vi "GeoData.vi"() -> ()   [LabVIEW 2017] (continued)
H1\n66625\t20177\tTopeka\tKS\tShawnee County\tH1\n66409\t20177\tBerryton\tKS\tShawnee County\tH1\n66536\t20177\tSaint marys\tKS\tShawnee County\tH1\n66524\t20177\tOverbrook\tKS\tShawnee County\tH1\n66614\t20177\tTopeka\tKS\tShawnee County\tH1\n66636\t20177\tTopeka\tKS\tShawnee County\tH1\n66667\t20177\tTopeka\tKS\tShawnee County\tH1\n66624\t20177\tTopeka\tKS\tShawnee County\tH1\n66420\t20177\tDover\tKS\tShawnee County\tH1\n66609\t20177\tTopeka\tKS\tShawnee County\tH1\n66615\t20177\tTopeka\tKS\tShawnee County\tH1\n66603\t20177\tTopeka\tKS\tShawnee County\tH1\n66546\t20177\tWakarusa\tKS\tShawnee County\tH1\n66647\t20177\tTopeka\tKS\tShawnee County\tH1\n66542\t20177\tTecumseh\tKS\tShawnee County\tH1\n66608\t20177\tTopeka\tKS\tShawnee County\tH1\n66612\t20177\tTopeka\tKS\tShawnee County\tH1\n66621\t20177\tTopeka\tKS\tShawnee County\tH1\n66620\t20177\tTopeka\tKS\tShawnee County\tH1\n66626\t20177\tTopeka\tKS\tShawnee County\tH1\n66533\t20177\tRossville\tKS\tShawnee County\tH1\n66604\t20177\tTopeka\tKS\tShawnee County\tH1\n66606\t20177\tTopeka\tKS\tShawnee County\tH1\n66675\t20177\tTopeka\tKS\tShawnee County\tH1\n66699\t20177\tTopeka\tKS\tShawnee County\tH1\n66402\t20177\tAuburn\tKS\tShawnee County\tH1\n66618\t20177\tTopeka\tKS\tShawnee County\tH1\n66607\t20177\tTopeka\tKS\tShawnee County\tH1\n66616\t20177\tTopeka\tKS\tShawnee County\tH1\n66683\t20177\tTopeka\tKS\tShawnee County\tH1\n66629\t20177\tTopeka\tKS\tShawnee County\tH1\n66622\t20177\tTopeka\tKS\tShawnee County\tH1\n67757\t20179\tSelden\tKS\tSheridan County\tH1\n67738\t20179\tGrinnell\tKS\tSheridan County\tH1\n67740\t20179\tHoxie\tKS\tSheridan County\tH1\n67753\t20179\tRexford\tKS\tSheridan County\tH1\n67732\t20181\tBrewster\tKS\tSherman County\tH1\n67741\t20181\tKanorado\tKS\tSherman County\tH1\n67735\t20181\tGoodland\tKS\tSherman County\tH1\n67733\t20181\tEdson\tKS\tSherman County\tH1\n67762\t20181\tWeskan\tKS\tSherman County\tH1\n66967\t20183\tSmith center\tKS\tSmith County\tH1\n67474\t20183\tPortis\tKS\tSmith County\tH1\n66941\t20183\tEsbon\tKS\tSmith County\tH1\n66952\t20183\tLebanon\tKS\tSmith County\tH1\n66951\t20183\tKensington\tKS\tSmith County\tH1\n66932\t20183\tAthol\tKS\tSmith County\tH1\n67628\t20183\tCedar\tKS\tSmith County\tH1\n67437\t20183\tDowns\tKS\tSmith County\tH1\n67638\t20183\tGaylord\tKS\tSmith County\tH1\n67526\t20185\tEllinwood\tKS\tStafford County\tH1\n67578\t20185\tStafford\tKS\tStafford County\tH1\n67545\t20185\tHudson\tKS\tStafford County\tH1\n67576\t20185\tSt john\tKS\tStafford County\tH1\n67530\t20185\tGreat bend\tKS\tStafford County\tH1\n67557\t20185\tMacksville\tKS\tStafford County\tH1\n67583\t20185\tTuron\tKS\tStafford County\tH1\n67855\t20187\tJohnson\tKS\tStanton County\tH1\n67862\t20187\tManter\tKS\tStanton County\tH1\n67880\t20187\tUlysses\tKS\tStanton County\tH1\n67878\t20187\tSyracuse\tKS\tStanton County\tH1\n67951\t20189\tHugoton\tKS\tStevens County\tH1\n67954\t20189\tRolla\tKS\tStevens County\tH1\n67953\t20189\tRichfield\tKS\tStevens County\tH1\n67952\t20189\tMoscow\tKS\tStevens County\tH1\n67026\t20191\tClearwater\tKS\tSumner County\tH1\n67022\t20191\tCaldwell\tKS\tSumner County\tH1\n67119\t20191\tOxford\tKS\tSumner County\tH1\n67110\t20191\tMulvane\tKS\tSumner County\tH1\n67049\t20191\tFreeport\tKS\tSumner County\tH1\n67152\t20191\tWellington\tKS\tSumner County\tH1\n67051\t20191\tGeuda springs\tKS\tSumner County\tH1\n67013\t20191\tBelle plaine\tKS\tSumner County\tH1\n67031\t20191\tConway springs\tKS\tSumner County\tH1\n67004\t20191\tArgonia\tKS\tSumner County\tH1\n67140\t20191\tSouth haven\tKS\tSumner County\tH1\n67120\t20191\tPeck\tKS\tSumner County\tH1\n67105\t20191\tMilan\tKS\tSumner County\tH1\n67146\t20191\tUdall\tKS\tSumner County\tH1\n67018\t20191\tBluff city\tKS\tSumner County\tH1\n67106\t20191\tMilton\tKS\tSumner County\tH1\n67103\t20191\tMayfield\tKS\tSumner County\tH1\n67118\t20191\tNorwich\tKS\tSumner County\tH1\n67748\t20193\tOakley\tKS\tThomas County\tH1\n67757\t20193\tSelden\tKS\tThomas County\tH1\n67732\t20193\tBrewster\tKS\tThomas County\tH1\n67764\t20193\tWinona\tKS\tThomas County\tH1\n67743\t20193\tLevant\tKS\tThomas County\tH1\n67747\t20193\tMonument\tKS\tThomas County\tH1\n67701\t20193\tColby\tKS\tThomas County\tH1\n67734\t20193\tGem\tKS\tThomas County\tH1\n67753\t20193\tRexford\tKS\tThomas County\tH1\n67656\t20195\tOgallah\tKS\tTrego County\tH1\n67752\t20195\tQuinter\tKS\tTrego County\tH1\n67584\t20195\tUtica\tKS\tTrego County\tH1\n67572\t20195\tRansom\tKS\tTrego County\tH1\n67672\t20195\tWakeeney\tKS\tTrego County\tH1\n67521\t20195\tBrownell\tKS\tTrego County\tH1\n67637\t20195\tEllis\tKS\tTrego County\tH1\n67631\t20195\tCollyer\tKS\tTrego County\tH1\n66431\t20197\tHarveyville\tKS\tWabaunsee County\tH1\n66610\t20197\tTopeka\tKS\tWabaunsee County\tH1\n66401\t20197\tAlma\tKS\tWabaunsee County\tH1\n66547\t20197\tWamego\tKS\tWabaunsee County\tH1\n66834\t20197\tAlta vista\tKS\tWabaunsee County\tH1\n66501\t20197\tMc farland\tKS\tWabaunsee County\tH1\n66502\t20197\tManhattan\tKS\tWabaunsee County\tH1\n66413\t20197\tBurlingame\tKS\tWabaunsee County\tH1\n66536\t20197\tSaint marys\tKS\tWabaunsee County\tH1\n66614\t20197\tTopeka\tKS\tWabaunsee County\tH1\n66407\t20197\tBelvue\tKS\tWabaunsee County\tH1\n66846\t20197\tCouncil grove\tKS\tWabaunsee County\tH1\n66615\t20197\tTopeka\tKS\tWabaunsee County\tH1\n66526\t20197\tPaxico\tKS\tWabaunsee County\tH1\n66423\t20197\tEskridge\tKS\tWabaunsee County\tH1\n66507\t20197\tMaple hill\tKS\tWabaunsee County\tH1\n67861\t20199\tLeoti\tKS\tWallace County\tH1\n67758\t20199\tSharon springs\tKS\tWallace County\tH1\n67761\t20199\tWallace\tKS\tWallace County\tH1\n67762\t20199\tWeskan\tKS\tWallace County\tH1\n66943\t20201\tGreenleaf\tKS\tWashington County\tH1\n66953\t20201\tLinn\tKS\tWashington County\tH1\n66933\t20201\tBarnes\tKS\tWashington County\tH1\n66946\t20201\tHollenberg\tKS\tWashington County\tH1\n66548\t20201\tWaterville\tKS\tWashington County\tH1\n66955\t20201\tMahaska\tKS\tWashington County\tH1\n66960\t20201\tNarka\tKS\tWashington County\tH1\n66945\t20201\tHanover\tKS\tWashington County\tH1\n66937\t20201\tClifton\tKS\tWashington County\tH1\n66412\t20201\tBremen\tKS\tWashington County\tH1\n66968\t20201\tWashington\tKS\tWashington County\tH1\n66958\t20201\tMorrowville\tKS\tWashington County\tH1\n66962\t20201\tPalmer\tKS\tWashington County\tH1\n66938\t20201\tClyde\tKS\tWashington County\tH1\n66944\t20201\tHaddam\tKS\tWashington County\tH1\n67861\t20203\tLeoti\tKS\tWichita County\tH1\n67863\t20203\tMarienthal\tKS\tWichita County\tH1\n66736\t20205\tFredonia\tKS\tWilson County\tH1\n66776\t20205\tThayer\tKS\tWilson County\tH1\n66757\t20205\tNeodesha\tKS\tWilson County\tH1\n66714\t20205\tBenedict\tKS\tWilson County\tH1\n66717\t20205\tBuffalo\tKS\tWilson County\tH1\n67047\t20205\tFall river\tKS\tWilson County\tH1\n66710\t20205\tAltoona\tKS\tWilson County\tH1\n66777\t20205\tToronto\tKS\tWilson County\tH1\n67335\t20205\tCherryvale\tKS\tWilson County\tH1\n66720\t20205\tChanute\tKS\tWilson County\tH1\n66749\t20207\tIola\tKS\tWoodson County\tH1\n66870\t20207\tVirgil\tKS\tWoodson County\tH1\n66783\t20207\tYates center\tKS\tWoodson County\tH1\n66736\t20207\tFredonia\tKS\tWoodson County\tH1\n66761\t20207\tPiqua\tKS\tWoodson County\tH1\n66748\t20207\tHumboldt\tKS\tWoodson County\tH1\n66852\t20207\tGridley\tKS\tWoodson County\tH1\n66758\t20207\tNeosho falls\tKS\tWoodson County\tH1\n66717\t20207\tBuffalo\tKS\tWoodson County\tH1\n66777\t20207\tToronto\tKS\tWoodson County\tH1\n66115\t20209\tKansas city\tKS\tWyandotte County\tH6\n66104\t20209\tKansas city\tKS\tWyandotte County\tH6\n66103\t20209\tKansas city\tKS\tWyandotte County\tH6\n66117\t20209\tKansas city\tKS\tWyandotte County\tH6\n66106\t20209\tKansas city\tKS\tWyandotte County\tH6\n66216\t20209\tShawnee\tKS\tWyandotte County\tH6\n66119\t20209\tKansas city\tKS\tWyandotte County\tH6\n66217\t20209\tShawnee\tKS\tWyandotte County\tH6\n66102\t20209\tKansas city\tKS\tWyandotte County\tH6\n66048\t20209\tLeavenworth\tKS\tWyandotte County\tH6\n66007\t20209\tBasehor\tKS\tWyandotte County\tH6\n66118\t20209\tKansas city\tKS\tWyandotte County\tH6\n66112\t20209\tKansas city\tKS\tWyandotte County\tH6\n66160\t20209\tKansas city\tKS\tWyandotte County\tH6\n66012\t20209\tBonner springs\tKS\tWyandotte County\tH6\n66109\t20209\tKansas city\tKS\tWyandotte County\tH6\n66111\t20209\tKansas city\tKS\tWyandotte County\tH6\n66101\t20209\tKansas city\tKS\tWyandotte County\tH6\n66105\t20209\tKansas city\tKS\tWyandotte County\tH6\n42129\t21001\tEdmonton\tKY\tAdair County\tH1\n42642\t21001\tRussell springs\tKY\tAdair County\tH1\n42728\t21001\tColumbia\tKY\tAdair County\tH1\n42715\t21001\tBreeding\tKY\tAdair County\tH1\n42741\t21001\tGlens fork\tKY\tAdair County\tH1\n42539\t21001\tLiberty\tKY\tAdair County\tH1\n42743\t21001\tGreensburg\tKY\tAdair County\tH1\n42742\t21001\tGradyville\tKY\tAdair County\tH1\n42733\t21001\tElk horn\tKY\tAdair County\tH1\n42718\t21001\tCampbellsville\tKY\tAdair County\tH1\n42753\t21001\tKnifley\tKY\tAdair County\tH1\n42528\t21001\tDunnville\tKY\tAdair County\tH1\n42720\t21001\tCane valley\tKY\tAdair County\tH1\n42133\t21003\tFountain run\tKY\tAllen County\tH1\n42134\t21003\tFranklin\tKY\tAllen County\tH1\n42122\t21003\tAlvaton\tKY\tAllen County\tH1\n42164\t21003\tScottsville\tKY\tAllen County\tH1\n42153\t21003\tHolland\tKY\tAllen County\tH1\n42120\t21003\tAdolphus\tKY\tAllen County\tH1\n40046\t21005\tMount eden\tKY\tAnderson County\tH1\n40012\t21005\tChaplin\tKY\tAnderson County\tH1\n40078\t21005\tWillisburg\tKY\tAnderson County\tH1\n40601\t21005\tFrankfort\tKY\tAnderson County\tH1\n40342\t21005\tLawrenceburg\tKY\tAnderson County\tH1\n40076\t21005\tWaddy\tKY\tAnderson County\tH1\n40372\t21005\tSalvisa\tKY\tAnderson County\tH1\n42024\t21007\tBarlow\tKY\tBallard County\tH1\n42053\t21007\tKevil\tKY\tBallard County\tH1\n42087\t21007\tWickliffe\tKY\tBallard County\tH1\n42022\t21007\tBandana\tKY\tBallard County\tH1\n42056\t21007\tLa center\tKY\tBallard County\tH1\n42060\t21007\tLovelaceville\tKY\tBallard County\tH1\n42133\t21009\tFountain run\tKY\tBarren County\tH1\n42131\t21009\tEtoile\tKY\tBarren County\tH1\n42171\t21009\tSmiths grove\tKY\tBarren County\tH1\n42166\t21009\tSummer shade\tKY\tBarren County\tH1\n42749\t21009\tHorse cave\tKY\tBarren County\tH1\n42152\t21009\tHiseville\tKY\tBarren County\tH1\n42123\t21009\tAustin\tKY\tBarren County\tH1\n42130\t21009\tEighty eight\tKY\tBarren County\tH1\n42127\t21009\tCave city\tKY\tBarren County\tH1\n42157\t21009\tMount hermon\tKY\tBarren County\tH1\n42154\t21009\tKnob lick\tKY\tBarren County\tH1\n42141\t21009\tGlasgow\tKY\tBarren County\tH1\n42156\t21009\tLucas\tKY\tBarren County\tH1\n42160\t21009\tPark city\tKY\tBarren County\tH1\n42746\t21009\tHardyville\tKY\tBarren County\tH1\n40358\t21011\tOlympia\tKY\tBath County\tH1\n40311\t21011\tCarlisle\tKY\tBath County\tH1\n40353\t21011\tMount sterling\tKY\tBath County\tH1\n40346\t21011\tMeans\tKY\tBath County\tH1\n40334\t21011\tHope\tKY\tBath County\tH1\n40351\t21011\tMorehead\tKY\tBath County\tH1\n41041\t21011\tFlemingsburg\tKY\tBath County\tH1\n40371\t21011\tSalt lick\tKY\tBath County\tH1\n40360\t21011\tOwingsville\tKY\tBath County\tH1\n40374\t21011\tSharpsburg\tKY\tBath County\tH1\n40322\t21011\tFrenchburg\tKY\tBath County\tH1\n40958\t21013\tKettle island\tKY\tBell County\tH1\n40930\t21013\tDewitt\tKY\tBell County\tH1\n40977\t21013\tPineville\tKY\tBell County\tH1\n40955\t21013\tIngram\tKY\tBell County\tH1\n40845\t21013\tHulen\tKY\tBell County\tH1\n40856\t21013\tMiracle\tKY\tBell County\tH1\n40939\t21013\tFourmile\tKY\tBell County\tH1\n40988\t21013\tStoney fork\tKY\tBell County\tH1\n40813\t21013\tCalvin\tKY\tBell County\tH1\n40902\t21013\tArjay\tKY\tBell County\tH1\n40965\t21013\tMiddlesboro\tKY\tBell County\tH1\n40913\t21013\tBeverly\tKY\tBell County\tH1\n40940\t21013\tFrakes\tKY\tBell County\tH1\n41048\t21015\tHebron\tKY\tBoone County\tH1\n45275\t21015\tCincinnati\tKY\tBoone County\tH1\n41025\t21015\tErlanger\tKY\tBoone County\tH1\n41091\t21015\tUnion\tKY\tBoone County\tH1\n41092\t21015\tVerona\tKY\tBoone County\tH1\n41005\t21015\tBurlington\tKY\tBoone County\tH1\n41018\t21015\tErlanger\tKY\tBoone County\tH1\n41030\t21015\tCrittenden\tKY\tBoone County\tH1\n41042\t21015\tFlorence\tKY\tBoone County\tH1\n41094\t21015\tWalton\tKY\tBoone County\tH1\n41080\t21015\tPetersburg\tKY\tBoone County\tH1\n41051\t21015\tIndependence\tKY\tBoone County\tH1\n41022\t21015\tFlorence\tKY\tBoone County\tH1\n40311\t21017\tCarlisle\tKY\tBourbon County\tH1\n41031\t21017\tCynthiana\tKY\tBourbon County\tH1\n40353\t21017\tMount sterling\tKY\tBourbon County\tH1\n40357\t21017\tNorth middletown\tKY\tBourbon County\tH1\n40324\t21017\tGeorgetown\tKY\tBourbon County\tH1\n40511\t21017\tLexington\tKY\tBourbon County\tH1\n40361\t21017\tParis\tKY\tBourbon County\tH1\n40516\t21017\tLexington\tKY\tBourbon County\tH1\n40348\t21017\tMillersburg\tKY\tBourbon County\tH1\n40374\t21017\tSharpsburg\tKY\tBourbon County\tH1\n41102\t21019\tAshland\tKY\tBoyd County\tH1\n41132\t21019\tDenton\tKY\tBoyd County\tH1\n41101\t21019\tAshland\tKY\tBoyd County\tH1\n41168\t21019\tRush\tKY\tBoyd County\tH1\n41129\t21019\tCatlettsburg\tKY\tBoyd County\tH1\n41230\t21019\tLouisa\tKY\tBoyd County\tH1\n41105\t21019\tAshland\tKY\tBoyd County\tH1\n40468\t21021\tPerryville\tKY\tBoyle County\tH1\n40464\t21021\tParksville\tKY\tBoyle County\tH1\n40440\t21021\tJunction city\tKY\tBoyle County\tH1\n40422\t21021\tDanville\tKY\tBoyle County\tH1\n40452\t21021\tMitchellsburg\tKY\tBoyle County\tH1\n40330\t21021\tHarrodsburg\tKY\tBoyle County\tH1\n40328\t21021\tGravel switch\tKY\tBoyle County\tH1\n41043\t21023\tFoster\tKY\tBracken County\tH1\n41044\t21023\tGermantown\tKY\tBracken County\tH1\n41002\t21023\tAugusta\tKY\tBracken County\tH1\n41034\t21023\tDover\tKY\tBracken County\tH1\n41004\t21023\tBrooksville\tKY\tBracken County\tH1\n41064\t21023\tMount olivet\tKY\tBracken County\tH1\n41040\t21023\tFalmouth\tKY\tBracken County\tH1\n41061\t21023\tMilford\tKY\tBracken County\tH1\n41339\t21025\tJackson\tKY\tBreathitt County\tH1\n41721\t21025\tBuckhorn\tKY\tBreathitt County\tH1\n41390\t21025\tWhick\tKY\tBreathitt County\tH1\n41745\t21025\tGays creek\tKY\tBreathitt County\tH1\n41311\t21025\tBeattyville\tKY\tBreathitt County\tH1\n41317\t21025\tClayhole\tKY\tBreathitt County\tH1\n41314\t21025\tBooneville\tKY\tBreathitt County\tH1\n41385\t21025\tVancleve\tKY\tBreathitt County\tH1\n41366\t21025\tRousseau\tKY\tBreathitt County\tH1\n41727\t21025\tChavies\tKY\tBreathitt County\tH1\n41301\t21025\tCampton\tKY\tBreathitt County\tH1\n41364\t21025\tRicetown\tKY\tBreathitt County\tH1\n41310\t21025\tBays\tKY\tBreathitt County\tH1\n41348\t21025\tLost creek\tKY\tBreathitt County\tH1\n40146\t21027\tIrvington\tKY\tBreckinridge County\tH1\n40161\t21027\tRhodelia\tKY\tBreckinridge County\tH1\n40157\t21027\tPayneville\tKY\tBreckinridge County\tH1\n42712\t21027\tBig clifty\tKY\tBreckinridge County\tH1\n40140\t21027\tGarfield\tKY\tBreckinridge County\tH1\n40170\t21027\tStephensport\tKY\tBreckinridge County\tH1\n40153\t21027\tMc quady\tKY\tBreckinridge County\tH1\n40111\t21027\tCloverport\tKY\tBreckinridge County\tH1\n40152\t21027\tMc daniels\tKY\tBreckinridge County\tH1\n40144\t21027\tHarned\tKY\tBreckinridge County\tH1\n42343\t21027\tFordsville\tKY\tBreckinridge County\tH1\n40175\t21027\tVine grove\tKY\tBreckinridge County\tH1\n42754\t21027\tLeitchfield\tKY\tBreckinridge County\tH1\n40171\t21027\tUnion star\tKY\tBreckinridge County\tH1\n40142\t21027\tGuston\tKY\tBreckinridge County\tH1\n40145\t21027\tHudson\tKY\tBreckinridge County\tH1\n40176\t21027\tWebster\tKY\tBreckinridge County\tH1\n40119\t21027\tFalls of rough\tKY\tBreckinridge County\tH1\n40115\t21027\tCuster\tKY\tBreckinridge County\tH1\n40143\t21027\tHardinsburg\tKY\tBreckinridge County\tH1\n40178\t21027\tWestview\tKY\tBreckinridge County\tH1\n40229\t21029\tLouisville\tKY\tBullitt County\tH1\n40207\t21029\tLouisville\tKY\tBullitt County\tH1\n40272\t21029\tLouisville\tKY\tBullitt County\tH1\n40166\t21029\tShepherdsville\tKY\tBullitt County\tH1\n40150\t21029\tLebanon junction\tKY\tBullitt County\tH1\n40177\t21029\tWest point\tKY\tBullitt County\tH1\n40110\t21029\tClermont\tKY\tBullitt County\tH1\n40047\t21029\tMount washington\tKY\tBullitt County\tH1\n40129\t21029\tHillview\tKY\tBullitt County\tH1\n40071\t21029\tTaylorsville\tKY\tBullitt County\tH1\n40165\t21029\tShepherdsville\tKY\tBullitt County\tH1\n40013\t21029\tCoxs creek\tKY\tBullitt County\tH1\n40109\t21029\tBrooks\tKY\tBullitt County\tH1\n40299\t21029\tLouisville\tKY\tBullitt County\tH1\n42101\t21031\tBowling green\tKY\tButler County\tH1\n42339\t21031\tDunmor\tKY\tButler County\tH1\n42288\t21031\tWoodbury\tKY\tButler County\tH1\n42721\t21031\tCaneyville\tKY\tButler County\tH1\n42219\t21031\tDunbar\tKY\tButler County\tH1\n42276\t21031\tRussellville\tKY\tButler County\tH1\n42256\t21031\tLewisburg\tKY\tButler County\tH1\n42333\t21031\tCromwell\tKY\tButler County\tH1\n42273\t21031\tRochester\tKY\tButler County\tH1\n42252\t21031\tJetson\tKY\tButler County\tH1\n42275\t21031\tRoundhill\tKY\tButler County\tH1\n42320\t21031\tBeaver dam\tKY\tButler County\tH1\n42201\t21031\tAberdeen\tKY\tButler County\tH1\n42261\t21031\tMorgantown\tKY\tButler County\tH1\n42211\t21033\tCadiz\tKY\tCaldwell County\tH1\n42411\t21033\tFredonia\tKY\tCaldwell County\tH1\n42445\t21033\tPrinceton\tKY\tCaldwell County\tH1\n42064\t21033\tMarion\tKY\tCaldwell County\tH1\n42408\t21033\tDawson springs\tKY\tCaldwell County\tH1\n42048\t21035\tHardin\tKY\tCalloway County\tH1\n42020\t21035\tAlmo\tKY\tCalloway County\tH1\n42054\t21035\tKirksey\tKY\tCalloway County\tH1\n42025\t21035\tBenton\tKY\tCalloway County\tH1\n42049\t21035\tHazel\tKY\tCalloway County\tH1\n42076\t21035\tNew concord\tKY\tCalloway County\tH1\n42071\t21035\tMurray\tKY\tCalloway County\tH1\n42040\t21035\tFarmington\tKY\tCalloway County\tH1\n42066\t21035\tMayfield\tKY\tCalloway County\tH1\n42036\t21035\tDexter\tKY\tCalloway County\tH1\n41074\t21037\tDayton\tKY\tCampbell County\tH1\n41071\t21037\tNewport\tKY\tCampbell County\tH1\n41076\t21037\tNewport\tKY\tCampbell County\tH1\n41001\t21037\tAlexandria\tKY\tCampbell County\tH1\n41059\t21037\tMelbourne\tKY\tCampbell County\tH1\n41075\t21037\tFort thomas\tKY\tCampbell County\tH1\n41007\t21037\tCalifornia\tKY\tCampbell County\tH1\n41085\t21037\tSilver grove\tKY\tCampbell County\tH1\n41072\t21037\tNewport\tKY\tCampbell County\tH1\n41099\t21037\tNewport\tKY\tCampbell County\tH1\n41006\t21037\tButler\tKY\tCampbell County\tH1\n41073\t21037\tBellevue\tKY\tCampbell County\tH1\n42039\t21039\tFancy farm\tKY\tCarlisle County\tH1\n42035\t21039\tCunningham\tKY\tCarlisle County\tH1\n42023\t21039\tBardwell\tKY\tCarlisle County\tH1\n42021\t21039\tArlington\tKY\tCarlisle County\tH1\n42069\t21039\tMelber\tKY\tCarlisle County\tH1\n40075\t21041\tTurners station\tKY\tCarroll County\tH1\n41045\t21041\tGhent\tKY\tCarroll County\tH1\n40006\t21041\tBedford\tKY\tCarroll County\tH1\n41098\t21041\tWorthville\tKY\tCarroll County\tH1\n41083\t21041\tSanders\tKY\tCarroll County\tH1\n41008\t21041\tCarrollton\tKY\tCarroll County\tH1\n40045\t21041\tMilton\tKY\tCarroll County\tH1\n40011\t21041\tCampbellsburg\tKY\tCarroll County\tH1\n41121\t21043\tArgillite\tKY\tCarter County\tH1\n41132\t21043\tDenton\tKY\tCarter County\tH1\n41143\t21043\tGrayson\tKY\tCarter County\tH1\n41171\t21043\tSandy hook\tKY\tCarter County\tH1\n40351\t21043\tMorehead\tKY\tCarter County\tH1\n41180\t21043\tWebbville\tKY\tCarter County\tH1\n41173\t21043\tSoldier\tKY\tCarter County\tH1\n41144\t21043\tGreenup\tKY\tCarter County\tH1\n41179\t21043\tVanceburg\tKY\tCarter County\tH1\n41168\t21043\tRush\tKY\tCarter County\tH1\n41141\t21043\tGarrison\tKY\tCarter County\tH1\n41142\t21043\tGrahn\tKY\tCarter County\tH1\n41164\t21043\tOlive hill\tKY\tCarter County\tH1\n41230\t21043\tLouisa\tKY\tCarter County\tH1\n41146\t21043\tHitchins\tKY\tCarter County\tH1\n40437\t21045\tHustonville\tKY\tCasey County\tH1\n40442\t21045\tKings mountain\tKY\tCasey County\tH1\n40009\t21045\tBradfordsville\tKY\tCasey County\tH1\n40484\t21045\tStanford\tKY\tCasey County\tH1\n40489\t21045\tWaynesburg\tKY\tCasey County\tH1\n42642\t21045\tRussell springs\tKY\tCasey County\tH1\n42541\t21045\tMiddleburg\tKY\tCasey County\tH1\n42728\t21045\tColumbia\tKY\tCasey County\tH1\n40464\t21045\tParksville\tKY\tCasey County\tH1\n42539\t21045\tLiberty\tKY\tCasey County\tH1\n42565\t21045\tWindsor\tKY\tCasey County\tH1\n42544\t21045\tNancy\tKY\tCasey County\tH1\n42566\t21045\tYosemite\tKY\tCasey County\tH1\n42733\t21045\tElk horn\tKY\tCasey County\tH1\n42553\t21045\tScience hill\tKY\tCasey County\tH1\n42516\t21045\tBethelridge\tKY\tCasey County\tH1\n40328\t21045\tGravel switch\tKY\tCasey County\tH1\n42528\t21045\tDunnville\tKY\tCasey County\tH1\n42215\t21047\tCerulean\tKY\tChristian County\tH1\n42266\t21047\tPembroke\tKY\tChristian County\tH1\n42236\t21047\tHerndon\tKY\tChristian County\tH1\n42232\t21047\tGracey\tKY\tChristian County\tH1\n42262\t21047\tOak grove\tKY\tChristian County\tH1\n42408\t21047\tDawson springs\tKY\tChristian County\tH1\n42254\t21047\tLa fayette\tKY\tChristian County\tH1\n42220\t21047\tElkton\tKY\tChristian County\tH1\n42217\t21047\tCrofton\tKY\tChristian County\tH1\n42453\t21047\tSaint charles\tKY\tChristian County\tH1\n42240\t21047\tHopkinsville\tKY\tChristian County\tH1\n42442\t21047\tNortonville\tKY\tChristian County\tH1\n42241\t21047\tHopkinsville\tKY\tChristian County\tH1\n42286\t21047\tTrenton\tKY\tChristian County\tH1\n42464\t21047\tWhite plains\tKY\tChristian County\tH1\n40353\t21049\tMount sterling\tKY\tClark County\tH1\n40509\t21049\tLexington\tKY\tClark County\tH1\n40312\t21049\tClay city\tKY\tClark County\tH1\n40391\t21049\tWinchester\tKY\tClark County\tH1\n40392\t21049\tWinchester\tKY\tClark County\tH1\n40515\t21049\tLexington\tKY\tClark County\tH1\n40914\t21051\tBig creek\tKY\tClay County\tH1\n40932\t21051\tFall rock\tKY\tClay County\tH1\n40951\t21051\tHima\tKY\tClay County\tH1\n40402\t21051\tAnnville\tKY\tClay County\tH1\n40906\t21051\tBarbourville\tKY\tClay County\tH1\n40972\t21051\tOneida\tKY\tClay County\tH1\n40941\t21051\tGarrard\tKY\tClay County\tH1\n40744\t21051\tLondon\tKY\tClay County\tH1\n40486\t21051\tTyner\tKY\tClay County\tH1\n40741\t21051\tLondon\tKY\tClay County\tH1\n40962\t21051\tManchester\tKY\tClay County\tH1\n40913\t21051\tBeverly\tKY\tClay County\tH1\n40944\t21051\tGoose rock\tKY\tClay County\tH1\n40831\t21051\tHarlan\tKY\tClay County\tH1\n40983\t21051\tSextons creek\tKY\tClay County\tH1\n42602\t21053\tAlbany\tKY\tClinton County\tH1\n42603\t21053\tAlpha\tKY\tClinton County\tH1\n42633\t21053\tMonticello\tKY\tClinton County\tH1\n42717\t21053\tBurkesville\tKY\tClinton County\tH1\n42038\t21055\tEddyville\tKY\tCrittenden County\tH1\n42459\t21055\tSturgis\tKY\tCrittenden County\tH1\n42411\t21055\tFredonia\tKY\tCrittenden County\tH1\n42078\t21055\tSalem\tKY\tCrittenden County\tH1\n42450\t21055\tProvidence\tKY\tCrittenden County\tH1\n42064\t21055\tMarion\tKY\tCrittenden County\tH1\n42037\t21055\tDycusburg\tKY\tCrittenden County\tH1\n42055\t21055\tKuttawa\tKY\tCrittenden County\tH1\n42033\t21055\tCrayne\tKY\tCrittenden County\tH1\n42129\t21057\tEdmonton\tKY\tCumberland County\tH1\n42715\t21057\tBreeding\tKY\tCumberland County\tH1\n42602\t21057\tAlbany\tKY\tCumberland County\tH1\n42759\t21057\tMarrowbone\tKY\tCumberland County\tH1\n42717\t21057\tBurkesville\tKY\tCumberland County\tH1\n42167\t21057\tTompkinsville\tKY\tCumberland County\tH1\n42348\t21059\tHawesville\tKY\tDaviess County\tH1\n42420\t21059\tHenderson\tKY\tDaviess County\tH1\n42302\t21059\tOwensboro\tKY\tDaviess County\tH1\n42327\t21059\tCalhoun\tKY\tDaviess County\tH1\n42301\t21059\tOwensboro\tKY\tDaviess County\tH1\n42351\t21059\tLewisport\tKY\tDaviess County\tH1\n42303\t21059\tOwensboro\tKY\tDaviess County\tH1\n42366\t21059\tPhilpot\tKY\tDaviess County\tH1\n42378\t21059\tWhitesville\tKY\tDaviess County\tH1\n42356\t21059\tMaple mount\tKY\tDaviess County\tH1\n42355\t21059\tMaceo\tKY\tDaviess County\tH1\n42304\t21059\tOwensboro\tKY\tDaviess County\tH1\n42376\t21059\tUtica\tKY\tDaviess County\tH1\n42101\t21061\tBowling green\tKY\tEdmonson County\tH1\n42171\t21061\tSmiths grove\tKY\tEdmonson County\tH1\n42210\t21061\tBrownsville\tKY\tEdmonson County\tH1\n42259\t21061\tMammoth cave\tKY\tEdmonson County\tH1\n42729\t21061\tCub run\tKY\tEdmonson County\tH1\n42721\t21061\tCaneyville\tKY\tEdmonson County\tH1\n42207\t21061\tBee spring\tKY\tEdmonson County\tH1\n42754\t21061\tLeitchfield\tKY\tEdmonson County\tH1\n42275\t21061\tRoundhill\tKY\tEdmonson County\tH1\n42285\t21061\tSweeden\tKY\tEdmonson County\tH1\n42163\t21061\tRocky hill\tKY\tEdmonson County\tH1\n42160\t21061\tPark city\tKY\tEdmonson County\tH1\n41171\t21063\tSandy hook\tKY\tElliott County\tH1\n41149\t21063\tIsonville\tKY\tElliott County\tH1\n40351\t21063\tMorehead\tKY\tElliott County\tH1\n41180\t21063\tWebbville\tKY\tElliott County\tH1\n41472\t21063\tWest liberty\tKY\tElliott County\tH1\n41164\t21063\tOlive hill\tKY\tElliott County\tH1\n40312\t21065\tClay city\tKY\tEstill County\tH1\n40380\t21065\tStanton\tKY\tEstill County\tH1\n40336\t21065\tIrvine\tKY\tEstill County\tH1\n40385\t21065\tWaco\tKY\tEstill County\tH1\n40472\t21065\tRavenna\tKY\tEstill County\tH1\n40503\t21067\tLexington\tKY\tFayette County\tH6\n40575\t21067\tLexington\tKY\tFayette County\tH6\n40512\t21067\tLexington\tKY\tFayette County\tH6\n40578\t21067\tLexington\tKY\tFayette County\tH6\n40509\t21067\tLexington\tKY\tFayette County\tH6\n40324\t21067\tGeorgetown\tKY\tFayette County\tH6\n40544\t21067\tLexington\tKY\tFayette County\tH6\n40536\t21067\tLexington\tKY\tFayette County\tH6\n40577\t21067\tLexington\tKY\tFayette County\tH6\n40580\t21067\tLexington\tKY\tFayette County\tH6\n40391\t21067\tWinchester\tKY\tFayette County\tH6\n40513\t21067\tLexington\tKY\tFayette County\tH6\n40533\t21067\tLexington\tKY\tFayette County\tH6\n40555\t21067\tLexington\tKY\tFayette County\tH6\n40591\t21067\tLexington\tKY\tFayette County\tH6\n40583\t21067\tLexington\tKY\tFayette County\tH6\n40576\t21067\tLexington\tKY\tFayette County\tH6\n40504\t21067\tLexington\tKY\tFayette County\tH6\n40511\t21067\tLexington\tKY\tFayette County\tH6\n40574\t21067\tLexington\tKY\tFayette County\tH6\n40582\t21067\tLexington\tKY\tFayette County\tH6\n40502\t21067\tLexington\tKY\tFayette County\tH6\n40361\t21067\tParis\tKY\tFayette County\tH6\n40517\t21067\tLexington\tKY\tFayette County\tH6\n40515\t21067\tLexington\tKY\tFayette County\tH6\n40516\t21067\tLexington\tKY\tFayette County\tH6\n40514\t21067\tLexington\tKY\tFayette County\tH6\n40588\t21067\tLexington\tKY\tFayette County\tH6\n40505\t21067\tLexington\tKY\tFayette County\tH6\n40356\t21067\tNicholasville\tKY\tFayette County\tH6\n40510\t21067\tLexington\tKY\tFayette County\tH6\n40524\t21067\tLexington\tKY\tFayette County\tH6\n40522\t21067\tLexington\tKY\tFayette County\tH6\n40506\t21067\tLexington\tKY\tFayette County\tH6\n40581\t21067\tLexington\tKY\tFayette County\tH6\n40508\t21067\tLexington\tKY\tFayette County\tH6\n40507\t21067\tLexington\tKY\tFayette County\tH6\n40523\t21067\tLexington\tKY\tFayette County\tH6\n40579\t21067\tLexington\tKY\tFayette County\tH6\n40526\t21067\tLexington\tKY\tFayette County\tH6\n41056\t21069\tMaysville\tKY\tFleming County\tH1\n41093\t21069\tWallingford\tKY\tFleming County\tH1\n41049\t21069\tHillsboro\tKY\tFleming County\tH1\n41081\t21069\tPlummers landing\tKY\tFleming County\tH1\n40351\t21069\tMorehead\tKY\tFleming County\tH1\n41055\t21069\tMayslick\tKY\tFleming County\tH1\n41039\t21069\tEwing\tKY\tFleming County\tH1\n41041\t21069\tFlemingsburg\tKY\tFleming County\tH1\n41037\t21069\tElizaville\tKY\tFleming County\tH1\n41642\t21071\tIvel\tKY\tFloyd County\tH1\n41612\t21071\tBypro\tKY\tFloyd County\tH1\n41651\t21071\tMinnie\tKY\tFloyd County\tH1\n41621\t21071\tDwale\tKY\tFloyd County\tH1\n41631\t21071\tGrethel\tKY\tFloyd County\tH1\n41606\t21071\tBevinsville\tKY\tFloyd County\tH1\n41647\t21071\tMc dowell\tKY\tFloyd County\tH1\n41650\t21071\tMelvin\tKY\tFloyd County\tH1\n41616\t21071\tDavid\tKY\tFloyd County\tH1\n41636\t21071\tHi hat\tKY\tFloyd County\tH1\n41602\t21071\tAuxier\tKY\tFloyd County\tH1\n41655\t21071\tPrinter\tKY\tFloyd County\tH1\n41265\t21071\tVan lear\tKY\tFloyd County\tH1\n41667\t21071\tWeeksbury\tKY\tFloyd County\tH1\n41645\t21071\tLangley\tKY\tFloyd County\tH1\n41622\t21071\tEastern\tKY\tFloyd County\tH1\n41663\t21071\tTram\tKY\tFloyd County\tH1\n41630\t21071\tGarrett\tKY\tFloyd County\tH1\n41653\t21071\tPrestonsburg\tKY\tFloyd County\tH1\n41619\t21071\tDrift\tKY\tFloyd County\tH1\n41604\t21071\tBeaver\tKY\tFloyd County\tH1\n41635\t21071\tHarold\tKY\tFloyd County\tH1\n41669\t21071\tWheelwright\tKY\tFloyd County\tH1\n41640\t21071\tHueysville\tKY\tFloyd County\tH1\n41666\t21071\tWayland\tKY\tFloyd County\tH1\n41643\t21071\tLackey\tKY\tFloyd County\tH1\n41659\t21071\tStanville\tKY\tFloyd County\tH1\n41607\t21071\tBlue river\tKY\tFloyd County\tH1\n41230\t21071\tLouisa\tKY\tFloyd County\tH1\n41603\t21071\tBanner\tKY\tFloyd County\tH1\n41605\t21071\tBetsy layne\tKY\tFloyd County\tH1\n41601\t21071\tAllen\tKY\tFloyd County\tH1\n41216\t21071\tEast point\tKY\tFloyd County\tH1\n41615\t21071\tDana\tKY\tFloyd County\tH1\n41660\t21071\tTeaberry\tKY\tFloyd County\tH1\n41649\t21071\tMartin\tKY\tFloyd County\tH1\n40621\t21073\tFrankfort\tKY\tFranklin County\tH1\n40347\t21073\tMidway\tKY\tFranklin County\tH1\n40602\t21073\tFrankfort\tKY\tFranklin County\tH1\n40379\t21073\tStamping ground\tKY\tFranklin County\tH1\n40601\t21073\tFrankfort\tKY\tFranklin County\tH1\n40342\t21073\tLawrenceburg\tKY\tFranklin County\tH1\n40076\t21073\tWaddy\tKY\tFranklin County\tH1\n40604\t21073\tFrankfort\tKY\tFranklin County\tH1\n40003\t21073\tBagdad\tKY\tFranklin County\tH1\n42041\t21075\tFulton\tKY\tFulton County\tH1\n42050\t21075\tHickman\tKY\tFulton County\tH1\n41045\t21077\tGhent\tKY\tGallatin County\tH1\n41046\t21077\tGlencoe\tKY\tGallatin County\tH1\n41083\t21077\tSanders\tKY\tGallatin County\tH1\n41086\t21077\tSparta\tKY\tGallatin County\tH1\n41092\t21077\tVerona\tKY\tGallatin County\tH1\n41030\t21077\tCrittenden\tKY\tGallatin County\tH1\n41095\t21077\tWarsaw\tKY\tGallatin County\tH1\n40403\t21079\tBerea\tKY\tGarrard County\tH1\n40484\t21079\tStanford\tKY\tGarrard County\tH1\n40444\t21079\tLancaster\tKY\tGarrard County\tH1\n40410\t21079\tBryantsville\tKY\tGarrard County\tH1\n40419\t21079\tCrab orchard\tKY\tGarrard County\tH1\n40461\t21079\tPaint lick\tKY\tGarrard County\tH1\n41097\t21081\tWilliamstown\tKY\tGrant County\tH1\n41046\t21081\tGlencoe\tKY\tGrant County\tH1\n41052\t21081\tJonesville\tKY\tGrant County\tH1\n41003\t21081\tBerry\tKY\tGrant County\tH1\n41092\t21081\tVerona\tKY\tGrant County\tH1\n41030\t21081\tCrittenden\tKY\tGrant County\tH1\n41035\t21081\tDry ridge\tKY\tGrant County\tH1\n41095\t21081\tWarsaw\tKY\tGrant County\tH1\n41010\t21081\tCorinth\tKY\tGrant County\tH1\n41040\t21081\tFalmouth\tKY\tGrant County\tH1\n42054\t21083\tKirksey\tKY\tGraves County\tH1\n42061\t21083\tLowes\tKY\tGraves County\tH1\n42041\t21083\tFulton\tKY\tGraves County\tH1\n42003\t21083\tPaducah\tKY\tGraves County\tH1\n42051\t21083\tHickory\tKY\tGraves County\tH1\n42088\t21083\tWingo\tKY\tGraves County\tH1\n42039\t21083\tFancy farm\tKY\tGraves County\tH1\n42085\t21083\tWater valley\tKY\tGraves County\tH1\n42025\t21083\tBenton\tKY\tGraves County\tH1\n42049\t21083\tHazel\tKY\tGraves County\tH1\n42079\t21083\tSedalia\tKY\tGraves County\tH1\n42035\t21083\tCunningham\tKY\tGraves County\tH1\n42063\t21083\tLynnville\tKY\tGraves County\tH1\n42027\t21083\tBoaz\tKY\tGraves County\tH1\n42071\t21083\tMurray\tKY\tGraves County\tH1\n42040\t21083\tFarmington\tKY\tGraves County\tH1\n42021\t21083\tArlington\tKY\tGraves County\tH1\n42082\t21083\tSymsonia\tKY\tGraves County\tH1\n42066\t21083\tMayfield\tKY\tGraves County\tH1\n42069\t21083\tMelber\tKY\tGraves County\tH1\n42726\t21085\tClarkson\tKY\tGrayson County\tH1\n42712\t21085\tBig clifty\tKY\tGrayson County\tH1\n42210\t21085\tBrownsville\tKY\tGrayson County\tH1\n42361\t21085\tOlaton\tKY\tGrayson County\tH1\n42762\t21085\tMillwood\tKY\tGrayson County\tH1\n42721\t21085\tCaneyville\tKY\tGrayson County\tH1\n42349\t21085\tHorse branch\tKY\tGrayson County\tH1\n42207\t21085\tBee spring\tKY\tGrayson County\tH1\n42754\t21085\tLeitchfield\tKY\tGrayson County\tH1\n40145\t21085\tHudson\tKY\tGrayson County\tH1\n42275\t21085\tRoundhill\tKY\tGrayson County\tH1\n40119\t21085\tFalls of rough\tKY\tGrayson County\tH1\n42261\t21085\tMorgantown\tKY\tGrayson County\tH1\n42716\t21087\tBuffalo\tKY\tGreen County\tH1\n40009\t21087\tBradfordsville\tKY\tGreen County\tH1\n42129\t21087\tEdmonton\tKY\tGreen County\tH1\n42728\t21087\tColumbia\tKY\tGreen County\tH1\n42757\t21087\tMagnolia\tKY\tGreen County\tH1\n42743\t21087\tGreensburg\tKY\tGreen County\tH1\n42764\t21087\tMount sherman\tKY\tGreen County\tH1\n42718\t21087\tCampbellsville\tKY\tGreen County\tH1\n42782\t21087\tSummersville\tKY\tGreen County\tH1\n42722\t21087\tCanmer\tKY\tGreen County\tH1\n42214\t21087\tCenter\tKY\tGreen County\tH1\n42746\t21087\tHardyville\tKY\tGreen County\tH1\n41102\t21089\tAshland\tKY\tGreenup County\tH1\n41121\t21089\tArgillite\tKY\tGreenup County\tH1\n41143\t21089\tGrayson\tKY\tGreenup County\tH1\n41169\t21089\tRussell\tKY\tGreenup County\tH1\n41139\t21089\tFlatwoods\tKY\tGreenup County\tH1\n41101\t21089\tAshland\tKY\tGreenup County\tH1\n41144\t21089\tGreenup\tKY\tGreenup County\tH1\n41174\t21089\tSouth portsmouth\tKY\tGreenup County\tH1\n41179\t21089\tVanceburg\tKY\tGreenup County\tH1\n41183\t21089\tWorthington\tKY\tGreenup County\tH1\n41175\t21089\tSouth shore\tKY\tGreenup County\tH1\n41141\t21089\tGarrison\tKY\tGreenup County\tH1\n41166\t21089\tQuincy\tKY\tGreenup County\tH1\n42348\t21091\tHawesville\tKY\tHancock County\tH1\n42343\t21091\tFordsville\tKY\tHancock County\tH1\n42364\t21091\tHawesville\tKY\tHancock County\tH1\n42351\t21091\tLewisport\tKY\tHancock County\tH1\n42366\t21091\tPhilpot\tKY\tHancock County\tH1\n42368\t21091\tReynolds station\tKY\tHancock County\tH1\n40051\t21093\tNew haven\tKY\tHardin County\tH1\n42712\t21093\tBig clifty\tKY\tHardin County\tH1\n40140\t21093\tGarfield\tKY\tHardin County\tH1\n42702\t21093\tElizabethtown\tKY\tHardin County\tH1\n40121\t21093\tFort knox\tKY\tHardin County\tH1\n42748\t21093\tHodgenville\tKY\tHardin County\tH1\n42740\t21093\tGlendale\tKY\tHardin County\tH1\n40159\t21093\tRadcliff\tKY\tHardin County\tH1\n40160\t21093\tRadcliff\tKY\tHardin County\tH1\n40150\t21093\tLebanon junction\tKY\tHardin County\tH1\n40177\t21093\tWest point\tKY\tHardin County\tH1\n42776\t21093\tSonora\tKY\tHardin County\tH1\n40162\t21093\tRineyville\tKY\tHardin County\tH1\n40175\t21093\tVine grove\tKY\tHardin County\tH1\n42788\t21093\tWhite mills\tKY\tHardin County\tH1\n42724\t21093\tCecilia\tKY\tHardin County\tH1\n42784\t21093\tUpton\tKY\tHardin County\tH1\n42701\t21093\tElizabethtown\tKY\tHardin County\tH1\n40122\t21093\tFort knox\tKY\tHardin County\tH1\n42732\t21093\tEastview\tKY\tHardin County\tH1\n40927\t21095\tClosplint\tKY\tHarlan County\tH1\n40854\t21095\tLoyall\tKY\tHarlan County\tH1\n40820\t21095\tCranks\tKY\tHarlan County\tH1\n40823\t21095\tCumberland\tKY\tHarlan County\tH1\n40819\t21095\tColdiron\tKY\tHarlan County\tH1\n40818\t21095\tCoalgood\tKY\tHarlan County\tH1\n40807\t21095\tBenham\tKY\tHarlan County\tH1\n40815\t21095\tCawood\tKY\tHarlan County\tH1\n40843\t21095\tHolmes mill\tKY\tHarlan County\tH1\n40829\t21095\tGrays knob\tKY\tHarlan County\tH1\n40849\t21095\tLejunior\tKY\tHarlan County\tH1\n40806\t21095\tBaxter\tKY\tHarlan County\tH1\n40824\t21095\tDayhoit\tKY\tHarlan County\tH1\n40855\t21095\tLynch\tKY\tHarlan County\tH1\n40962\t21095\tManchester\tKY\tHarlan County\tH1\n40828\t21095\tEvarts\tKY\tHarlan County\tH1\n40840\t21095\tHelton\tKY\tHarlan County\tH1\n40801\t21095\tAges brookside\tKY\tHarlan County\tH1\n40865\t21095\tPutney\tKY\tHarlan County\tH1\n40830\t21095\tGulston\tKY\tHarlan County\tH1\n40831\t21095\tHarlan\tKY\tHarlan County\tH1\n40810\t21095\tBledsoe\tKY\tHarlan County\tH1\n40808\t21095\tBig laurel\tKY\tHarlan County\tH1\n40863\t21095\tPathfork\tKY\tHarlan County\tH1\n40847\t21095\tKenvir\tKY\tHarlan County\tH1\n40870\t21095\tTotz\tKY\tHarlan County\tH1\n40873\t21095\tWallins creek\tKY\tHarlan County\tH1\n40964\t21095\tMary alice\tKY\tHarlan County\tH1\n40311\t21097\tCarlisle\tKY\tHarrison County\tH1\n41031\t21097\tCynthiana\tKY\tHarrison County\tH1\n40370\t21097\tSadieville\tKY\tHarrison County\tH1\n41003\t21097\tBerry\tKY\tHarrison County\tH1\n41064\t21097\tMount olivet\tKY\tHarrison County\tH1\n40361\t21097\tParis\tKY\tHarrison County\tH1\n41010\t21097\tCorinth\tKY\tHarrison County\tH1\n41040\t21097\tFalmouth\tKY\tHarrison County\tH1\n42729\t21099\tCub run\tKY\tHart County\tH1\n42749\t21099\tHorse cave\tKY\tHart County\tH1\n42757\t21099\tMagnolia\tKY\tHart County\tH1\n42765\t21099\tMunfordville\tKY\tHart County\tH1\n42127\t21099\tCave city\tKY\tHart County\tH1\n42764\t21099\tMount sherman\tKY\tHart County\tH1\n42782\t21099\tSummersville\tKY\tHart County\tH1\n42722\t21099\tCanmer\tKY\tHart County\tH1\n42784\t21099\tUpton\tKY\tHart County\tH1\n42713\t21099\tBonnieville\tKY\tHart County\tH1\n42746\t21099\tHardyville\tKY\tHart County\tH1\n42419\t21101\tHenderson\tKY\tHenderson County\tH1\n42457\t21101\tSmith mills\tKY\tHenderson County\tH1\n42452\t21101\tRobards\tKY\tHenderson County\tH1\n42420\t21101\tHenderson\tKY\tHenderson County\tH1\n42451\t21101\tReed\tKY\tHenderson County\tH1\n42301\t21101\tOwensboro\tKY\tHenderson County\tH1\n42462\t21101\tWaverly\tKY\tHenderson County\tH1\n42402\t21101\tBaskett\tKY\tHenderson County\tH1\n42461\t21101\tUniontown\tKY\tHenderson County\tH1\n42458\t21101\tSpottsville\tKY\tHenderson County\tH1\n42406\t21101\tCorydon\tKY\tHenderson County\tH1\n40019\t21103\tEminence\tKY\tHenry County\tH1\n40036\t21103\tLockport\tKY\tHenry County\tH1\n40075\t21103\tTurners station\tKY\tHenry County\tH1\n40058\t21103\tPort royal\tKY\tHenry County\tH1\n40006\t21103\tBedford\tKY\tHenry County\tH1\n40601\t21103\tFrankfort\tKY\tHenry County\tH1\n40050\t21103\tNew castle\tKY\tHenry County\tH1\n40057\t21103\tPleasureville\tKY\tHenry County\tH1\n40068\t21103\tSmithfield\tKY\tHenry County\tH1\n40031\t21103\tLa grange\tKY\tHenry County\tH1\n40011\t21103\tCampbellsburg\tKY\tHenry County\tH1\n40070\t21103\tSulphur\tKY\tHenry County\tH1\n40055\t21103\tPendleton\tKY\tHenry County\tH1\n40007\t21103\tBethlehem\tKY\tHenry County\tH1\n42041\t21105\tFulton\tKY\tHickman County\tH1\n42088\t21105\tWingo\tKY\tHickman County\tH1\n42039\t21105\tFancy farm\tKY\tHickman County\tH1\n42085\t21105\tWater valley\tKY\tHickman County\tH1\n42031\t21105\tClinton\tKY\tHickman County\tH1\n42032\t21105\tColumbus\tKY\tHickman County\tH1\n42021\t21105\tArlington\tKY\tHickman County\tH1\n42066\t21105\tMayfield\tKY\tHickman County\tH1\n42445\t21107\tPrinceton\tKY\tHopkins County\tH1\n42450\t21107\tProvidence\tKY\tHopkins County\tH1\n42410\t21107\tEarlington\tKY\tHopkins County\tH1\n42408\t21107\tDawson springs\tKY\tHopkins County\tH1\n42431\t21107\tMadisonville\tKY\tHopkins County\tH1\n42441\t21107\tNebo\tKY\tHopkins County\tH1\n42453\t21107\tSaint charles\tKY\tHopkins County\tH1\n42442\t21107\tNortonville\tKY\tHopkins County\tH1\n42436\t21107\tManitou\tKY\tHopkins County\tH1\n42440\t21107\tMortons gap\tKY\tHopkins County\tH1\n42413\t21107\tHanson\tKY\tHopkins County\tH1\n42456\t21107\tSlaughters\tKY\tHopkins County\tH1\n42464\t21107\tWhite plains\tKY\tHopkins County\tH1\n40481\t21109\tSandgap\tKY\tJackson County\tH1\n40402\t21109\tAnnville\tKY\tJackson County\tH1\n40486\t21109\tTyner\tKY\tJackson County\tH1\n40447\t21109\tMc kee\tKY\tJackson County\tH1\n40962\t21109\tManchester\tKY\tJackson County\tH1\n40434\t21109\tGray hawk\tKY\tJackson County\tH1\n40456\t21109\tMount vernon\tKY\tJackson County\tH1\n40445\t21109\tLivingston\tKY\tJackson County\tH1\n40269\t21111\tLouisville\tKY\tJefferson County\tH1\n40041\t21111\tMasonic home\tKY\tJefferson County\tH1\n40259\t21111\tLouisville\tKY\tJefferson County\tH1\n40280\t21111\tLouisville\tKY\tJefferson County\tH1\n40282\t21111\tLouisville\tKY\tJefferson County\tH1\n40229\t21111\tLouisville\tKY\tJefferson 
